vi "State Actor Destroy.vi"(7 "Self Actor in":refnum<class "Self Actor.lvclass">, 11 "Msging Self Actor State in":refnum<class "Msging Self Actor State.lvclass">) -> (0 "error out":errorcluster)   [LabVIEW 2021, in "LVCAM.lvlib" / "Msging Self Actor State.lvclass"]
uses:
  Msging Self Actor State.lvclass
  Self Actor/Self Actor.lvclass
  C:/PPLs/LabVIEW-Composed-Actor-Model-LVCAM/LabVIEW-Composed-Actor-Model-LVCAM/LVCAM/LVCAM/Actor/Actor.lvclass
  Msgs/Actor Destroy/Actor Destroy Msg Strategy/Actor Destroy Msg Strategy.lvclass
  C:/PPLs/LabVIEW-Composed-Actor-Model-LVCAM/LabVIEW-Composed-Actor-Model-LVCAM/LVCAM/LVCAM/Msg Strategy/Msg Strategy.lvclass
  Self Actor/Nest Msg Send.vi
  LVCAM.lvlib
  C:/PPLs/LabVIEW-Composed-Actor-Model-LVCAM/LabVIEW-Composed-Actor-Model-LVCAM/LVCAM/Msgs/Actor Create/Actor Create/Actor Create.lvclass
  C:/PPLs/LabVIEW-Composed-Actor-Model-LVCAM/LabVIEW-Composed-Actor-Model-LVCAM/LVCAM/Msgs/Actor Destroy/Actor Destroy/Actor Destroy.lvclass
  C:/PPLs/LabVIEW-Composed-Actor-Model-LVCAM/LabVIEW-Composed-Actor-Model-LVCAM/LVCAM/Msgs/Actor Last Ack/Actor Last Ack/Actor Last Ack.lvclass
  C:/PPLs/LabVIEW-Composed-Actor-Model-LVCAM/LabVIEW-Composed-Actor-Model-LVCAM/LVCAM/LVCAM/Self Actor/Self Actor.lvclass
  C:/PPLs/LabVIEW-Composed-Actor-Model-LVCAM/LabVIEW-Composed-Actor-Model-LVCAM/LVCAM/Msgs/Actor Destroy/Actor Destroy Msg Strategy/Actor Destroy Msg Strategy.lvclass
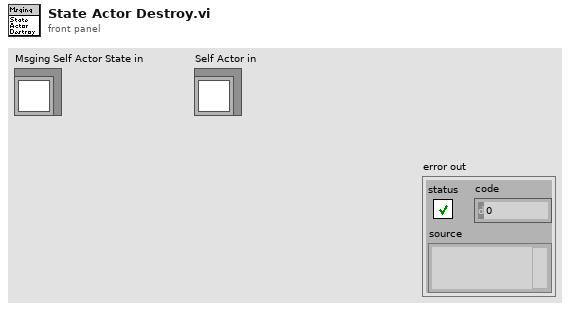
[diagram p1: front panel]
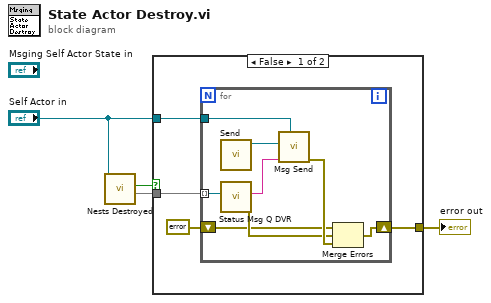
[diagram p0: block diagram]
diagram:
  n1 = call "Nests Destroyed.vi"("Self Actor in"="Self Actor in") -> ("Nest Msg Q DVRs"=w2:set{refnum<data-value>}, "Nests Destroyed?"=w3:bool)  [unwired: 9 in]
  n2 = case shown="False" w3 {
    tunnel: w2 -> [w8 _]
    tunnel: [w7 _] -> w4
    tunnel: "Self Actor in" -> [w5 _]
    frame False {
      n3 = for {
        tunnel: w8 -> [w12] mode=indexing
        shift-right: [w16] -> w7
        shift-left: errorcluster {"status"=FALSE, "code"=0, "source"=""} ("error out") -> [w9]
        tunnel: w5 -> [w13]
        n4 = call "Send.vi"() -> ("Actor Destroy Msg Strategy out"=w14:refnum<class "Actor Destroy Msg Strategy.lvclass">)  [unwired: 11 in]
        n5 = call "Status Msg Q DVR.vi"("Msg Q DVR"=w12) -> ("error out"=w10:errorcluster, "Msg Q DVR Alias"=w11:string)  [unwired: 9 in]
        n6 = call-poly "Msg Send.vi"("Actor"=w13, "Alias"=w11, "Msg"=w14) -> ("error out"=w15:errorcluster)  [unwired: 8 in]
        n7 = Merge Errors(w9, w10, w15) -> (w16:errorcluster)
      }
    }
    frame True {
      # "there exist no Nest Actors to be destroyed, do nothing"
    }
  }
  "error out" <- w4
